vi "Config.vi"(8 "error in (no error)":errorcluster, 10 "Setting":variant, 11 "KE65XX DMM in":refnum<class "Keithley 65XX DMM.lvclass">) -> (0 "error out":errorcluster, 3 "KE65XX DMM out":refnum<class "Keithley 65XX DMM.lvclass">)   [LabVIEW 2025, in "DMM.lvlib" / "Keithley 65XX DMM.lvclass"]
uses:
  Keithley 65XX DMM.lvclass
  Keithley 65XX DMM.lvclass/Keithley 65XX DMM.ctl
  <instrlib>/Keithley 65XX/Drivers/Keithley DMM6500 DAQ6500 Series.lvlib
  DMM configuration/DMM configuration.lvclass
  DMM Channel/DMM Channel.lvclass
  Users/Public/Documents/Sandia National Labs/TSS Plugin/Abstract Engine.lvlibp/Plugin/Abstract/Channel configuration/Channel configuration.lvclass
  Users/Public/Documents/Sandia National Labs/TSS Plugin/Abstract Engine.lvlibp/Plugin/Abstract/Abstract Instrument/Channel.ctl
  Users/Public/Documents/Sandia National Labs/TSS Plugin/Abstract Engine.lvlibp/Plugin/Abstract/Abstract Instrument/Abstract Instrument.lvclass
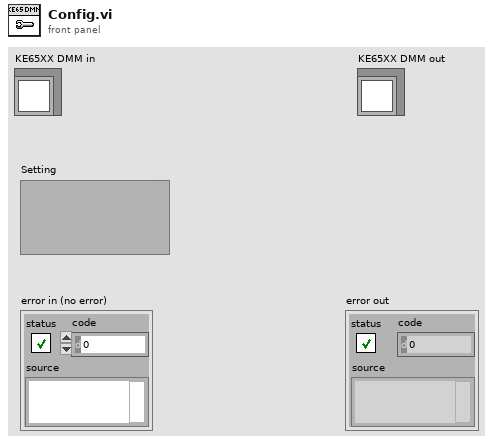
[diagram p1: front panel]
types:
  T1 = typedef "DMM.lvlib/DMM configuration.lvclass/DMM Setting.ctl" = cluster{"Function":string, "CurrentSource":string, "Resolution":string, "Range":dbl}
  T2 = typedef "Abstract Engine.lvlibp/Abstract Instrument.lvclass/Channel.ctl" = cluster{"Alias":string, "DataType":enum16{"Anaolg Input", "Waveform"}, "Unit":enum16{"---", "V", "A", "Ohm", "Hz", "uF", "degC", "deg"}, "Upper limit":dbl, "Lower limit":dbl, "Measurement":variant}
  T3 = typedef "Abstract Engine.lvlibp/Channel configuration.lvclass/Default Channel.ctl" = cluster{"Address":string, "SW Alias":string, "Enabled":bool, "Type":string, "Description":string}
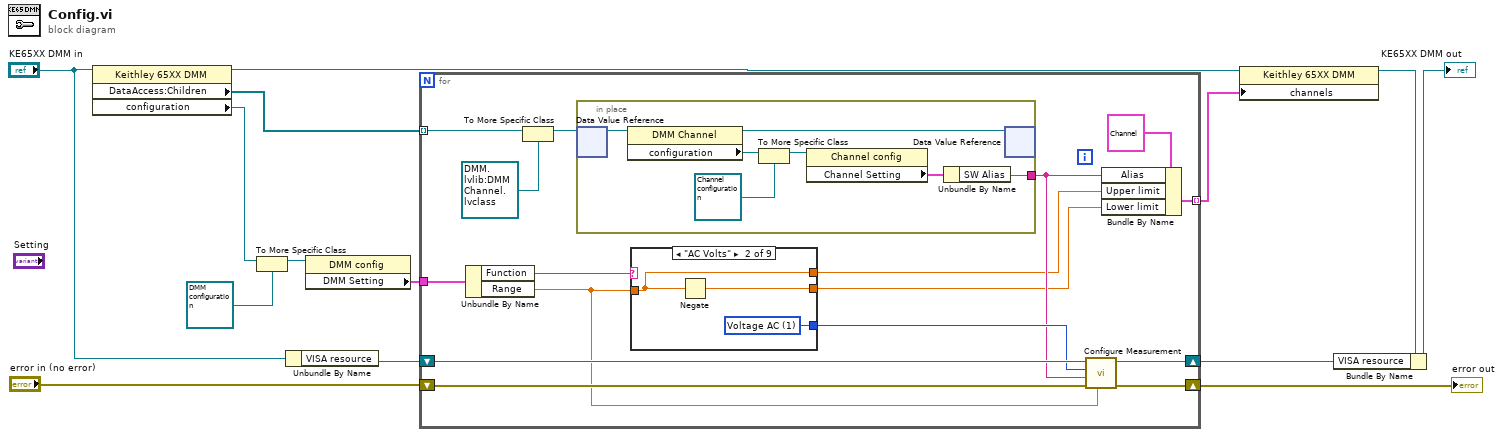
[diagram p0: block diagram]
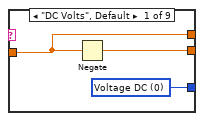
[diagram p2: hidden frame]
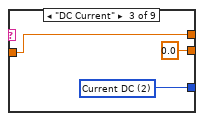
[diagram p3: hidden frame]
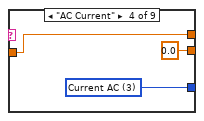
[diagram p4: hidden frame]
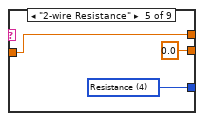
[diagram p5: hidden frame]
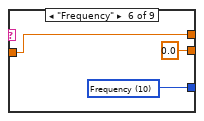
[diagram p6: hidden frame]
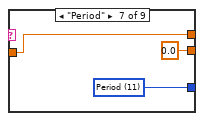
[diagram p7: hidden frame]
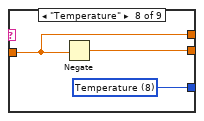
[diagram p8: hidden frame]
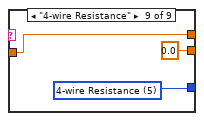
[diagram p9: hidden frame]
diagram:
  n1 = property class="Keithley 65XX DMM"(reference="KE65XX DMM in") -> (reference out=w11:refnum<class "Keithley 65XX DMM.lvclass">, "DataAccess:Children"=w8:refnum<data-value>[], "configuration"=w9:refnum<class "CEF_serializable configuration.lvclass">)  [unwired: 1 in, 1 out]
  n2 = To More Specific Class(target class=refnum<class "DMM configuration.lvclass"> refnum ("DMM.lvlib:DMM configuration.lvclass"), reference=w9) -> (specific class reference=w10:refnum<class "DMM configuration.lvclass">)  [unwired: 1 in, 1 out]
  n3 = Unbundle By Name("KE65XX DMM in") -> ("VISA resource"=w14:refnum<visa-resource-name>)
  n4 = property class="DMM config"(reference=w10) -> ("DMM Setting"=w5:T1)  [unwired: 1 in, 2 out]
  n5 = for {
    tunnel: w5 -> [w28]
    shift-right: [w29] -> w12
    shift-left: w14 -> [w30]
    tunnel: w8 -> [w25] mode=indexing
    shift-right: [w23] -> w7
    shift-left: "error in (no error)" -> [w22]
    tunnel: [w20] -> w1 mode=indexing
    n6 = Unbundle By Name(w28) -> ("Function"=w27:string, "Range"=w18:dbl)
    n7 = To More Specific Class(target class=refnum<data-value> refnum ("data value reference"), reference=w25) -> (specific class reference=w24:refnum<data-value>)  [unwired: 1 in, 1 out]
    n8 = in-place {
      in-place-border: [w33] -> w19
      n9 = in-place-dvr #1(w24) -> (w37:refnum<class "DMM Channel.lvclass">)  [unwired: 1 out]
      n10 = property class="DMM Channel"(reference=w37) -> (reference out=w36:refnum<class "DMM Channel.lvclass">, "configuration"=w35:refnum<class "CEF_serializable configuration.lvclass">)  [unwired: 1 in, 1 out]
      n11 = To More Specific Class(target class=refnum<class "Channel configuration.lvclass"> refnum ("Abstract Engine.lvlibp:Channel config"), reference=w35) -> (specific class reference=w34:refnum<class "Channel configuration.lvclass">)  [unwired: 1 in, 1 out]
      n12 = property class="Channel config"(reference=w34) -> ("Channel Setting"=w32:T3)  [unwired: 1 in, 2 out]
      n13 = Unbundle By Name(w32) -> ("SW Alias"=w33:string)
      n14 = in-place-dvr #1(w36) -> ()  [unwired: 2 out]
    }
    n15 = case shown="\"AC Volts\"" w27 {
      tunnel: [w40 w43 w46 w49 w52 w55 w58 w61 w64] -> w26
      tunnel: w18 -> [w39 w42 w45 w48 w51 w54 w57 w60 w63]
      tunnel: [w39 w42 w45 w48 w51 w54 w57 w60 w63] -> w17
      tunnel: [w38 w41 0.0 0.0 0.0 0.0 0.0 w59 0.0] -> w16
      frame "DC Volts", Default {
        w40 = 0 items=[" Voltage DC", "Voltage AC", "Current DC", "Current AC", "Resistance", "4-wire Resistance", "Diode", "Capacitance", "Temperature", "Continuity", "Frequency", "Period", "Voltage Ratio"] ("Function (0: Voltage DC)")
        n16 = Negate(x=w39) -> (-x=w38:dbl)
      }
      frame "AC Volts" {
        w43 = 1 items=[" Voltage DC", "Voltage AC", "Current DC", "Current AC", "Resistance", "4-wire Resistance", "Diode", "Capacitance", "Temperature", "Continuity", "Frequency", "Period", "Voltage Ratio"] ("Function (0: Voltage DC)")
        n17 = Negate(x=w42) -> (-x=w41:dbl)
      }
      frame "DC Current" {
        w46 = 2 items=[" Voltage DC", "Voltage AC", "Current DC", "Current AC", "Resistance", "4-wire Resistance", "Diode", "Capacitance", "Temperature", "Continuity", "Frequency", "Period", "Voltage Ratio"] ("Function (0: Voltage DC)")
      }
      frame "AC Current" {
        w49 = 3 items=[" Voltage DC", "Voltage AC", "Current DC", "Current AC", "Resistance", "4-wire Resistance", "Diode", "Capacitance", "Temperature", "Continuity", "Frequency", "Period", "Voltage Ratio"] ("Function (0: Voltage DC)")
      }
      frame "2-wire Resistance" {
        w52 = 4 items=[" Voltage DC", "Voltage AC", "Current DC", "Current AC", "Resistance", "4-wire Resistance", "Diode", "Capacitance", "Temperature", "Continuity", "Frequency", "Period", "Voltage Ratio"] ("Function (0: Voltage DC)")
      }
      frame "Frequency" {
        w55 = 10 items=[" Voltage DC", "Voltage AC", "Current DC", "Current AC", "Resistance", "4-wire Resistance", "Diode", "Capacitance", "Temperature", "Continuity", "Frequency", "Period", "Voltage Ratio"] ("Function (0: Voltage DC)")
      }
      frame "Period" {
        w58 = 11 items=[" Voltage DC", "Voltage AC", "Current DC", "Current AC", "Resistance", "4-wire Resistance", "Diode", "Capacitance", "Temperature", "Continuity", "Frequency", "Period", "Voltage Ratio"] ("Function (0: Voltage DC)")
      }
      frame "Temperature" {
        w61 = 8 items=[" Voltage DC", "Voltage AC", "Current DC", "Current AC", "Resistance", "4-wire Resistance", "Diode", "Capacitance", "Temperature", "Continuity", "Frequency", "Period", "Voltage Ratio"] ("Function (0: Voltage DC)")
        n18 = Negate(x=w60) -> (-x=w59:dbl)
      }
      frame "4-wire Resistance" {
        w64 = 5 items=[" Voltage DC", "Voltage AC", "Current DC", "Current AC", "Resistance", "4-wire Resistance", "Diode", "Capacitance", "Temperature", "Continuity", "Frequency", "Period", "Voltage Ratio"] ("Function (0: Voltage DC)")
      }
    }
    n19 = call <instrlib>:"Configure Measurement.vi"("Manual Range (0)"=w18, "error in (no error)"=w22, "Channel List(\"\")"=w19, "Function (0: Voltage DC)"=w26, "VISA resource name"=w30) -> ("error out"=w23:errorcluster, "VISA resource name out"=w29:refnum<visa-resource-name>)  [unwired: 5 in]
    n20 = Bundle By Name(cluster=T2 {"Alias"="ch0", "DataType"=enum."Anaolg Input", "Unit"=enum."V", "Upper limit"=10.0, "Lower limit"=-10.0, "Measurement"=variant} ("Channel"), "Alias"=w19, "Upper limit"=w17, "Lower limit"=w16) -> (w20:T2)
  }
  "error out" <- w7
  n21 = property class="Keithley 65XX DMM"(reference=w11, "channels"=w1) -> (reference out=w2:refnum<class "Keithley 65XX DMM.lvclass">)  [unwired: 1 in, 1 out]
  n22 = Bundle By Name(cluster=w2, "VISA resource"=w12) -> (→"KE65XX DMM out":refnum<class "Keithley 65XX DMM.lvclass">)
